vi "Android_Publisher_SM.vi"() -> ()   [LabVIEW 2015]
uses:
  <vilib>/daq.io/MQTT LabVIEW Client/Controls/Connection_Return_Codes.ctl
  Android_Data.ctl
  <vilib>/daq.io/MQTT LabVIEW Client/Controls/QoS.ctl
  <vilib>/daq.io/MQTT LabVIEW Client/Controls/Retain_Flag.ctl
  <vilib>/daq.io/MQTT LabVIEW Client/Controls/DUP_Flag.ctl
  Internet of Things Project/States.ctl
  <vilib>/Instr/_visa.llb/VISA Configure Serial Port (Instr).vi
  <vilib>/daq.io/MQTT LabVIEW Client/MQTT_Functions.lvlib
panel:
  in  "Data":T1={"VISA resource name"="ASRL1::INSTR", "baud rate (9600)"=19200, "Client ID"="myRIO", "Topic"="android", "MQTT Broker"={"address (IP)"="52.37.169.179", "port"=1883}, "Publish Meta"={"QoS"=enum."At most once", "Retain"=FALSE, "DUP"=FALSE}, "TCP connection ID "=refnum, "Session Status"=""}
  out "error out":errorcluster
  out "Session Status":string
  out "Published Data":string[][](array[string])
  in  "Stop Button":bool
  out "Connection Status":T5=enum."Connection refused: not authorized"
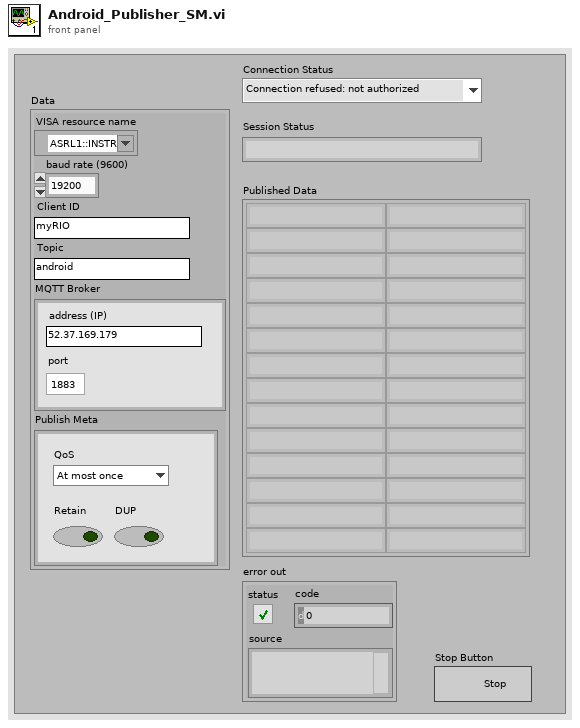
[diagram p1: front panel]
types:
  T1 = typedef "Android_Data.ctl" = cluster{"VISA resource name":refnum<visa-resource-name>, "baud rate (9600)":u32, "Client ID":string, "Topic":string, "MQTT Broker":cluster{"address (IP)":string, "port":u16}, "Publish Meta":cluster{"QoS":T2, "Retain":T3, "DUP":T4}, "TCP connection ID ":refnum<k5>, "Session Status":string}
  T2 = typedef "MQTT_Functions.lvlib/QoS.ctl" = enum8{"At most once", "At least once", "Exactly once", "Reserved"}
  T3 = typedef "MQTT_Functions.lvlib/Retain_Flag.ctl" = bool
  T4 = typedef "MQTT_Functions.lvlib/DUP_Flag.ctl" = bool
  T5 = typedef "MQTT_Functions.lvlib/Connection_Return_Codes.ctl" = enum16{"Connection accepted", "Connection refused: unacceptable protocol version", "Connection refused: identifier rejected", "Connection refused: Server unavailable", "Connection refused: bad user name or password", "Connection refused: not authorized"}
  T6 = typedef "States.ctl" = enum16{"Initialize", "TCP Connect", "Gather/Publish", "TCP Ping", "Exit/Disconnect"}
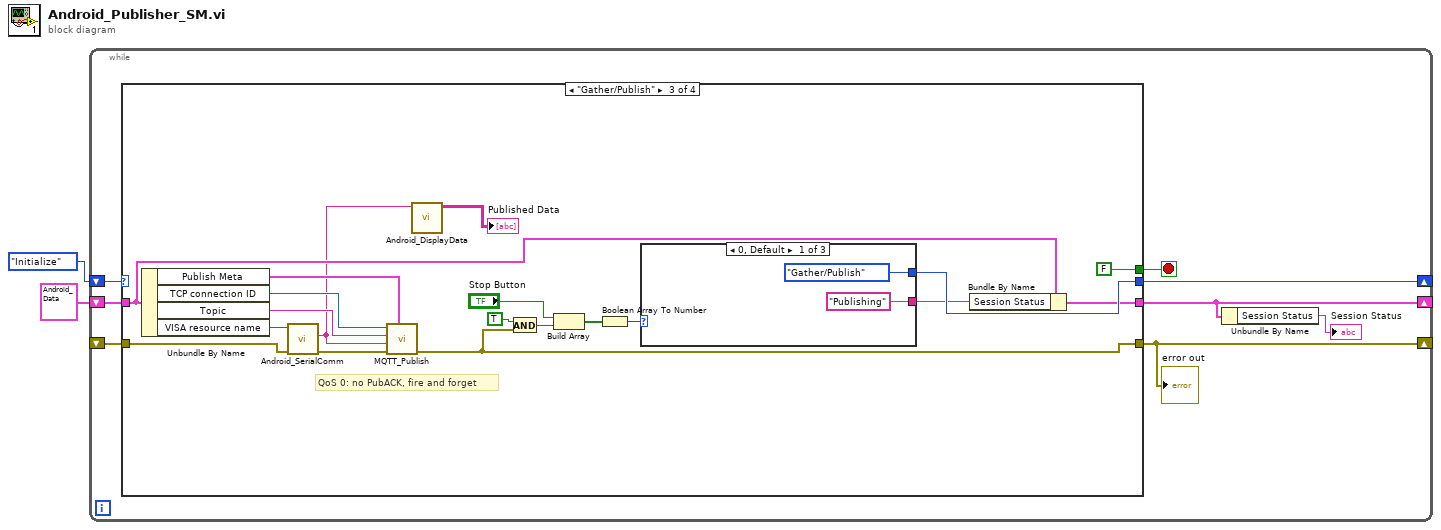
[diagram p0: block diagram]
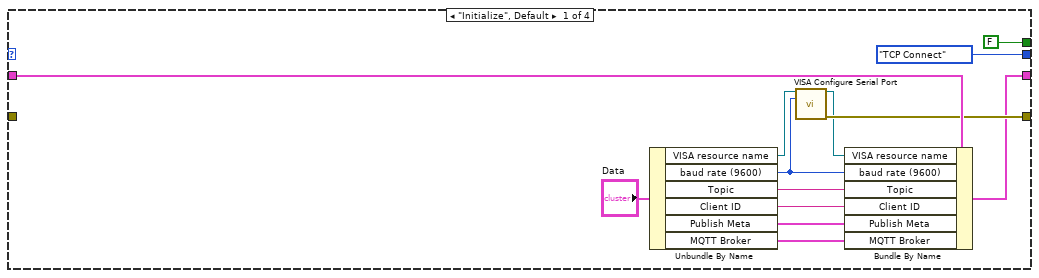
[diagram p2: hidden frame]
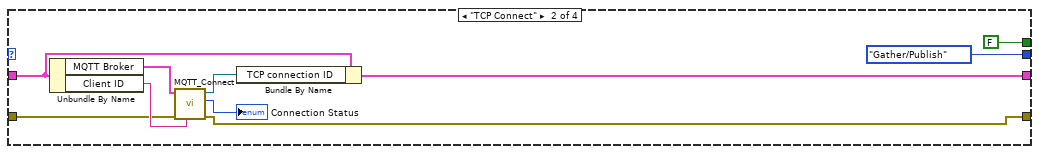
[diagram p3: hidden frame]
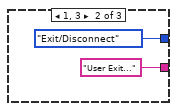
[diagram p4: hidden frame]
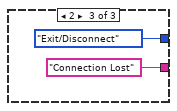
[diagram p5: hidden frame]
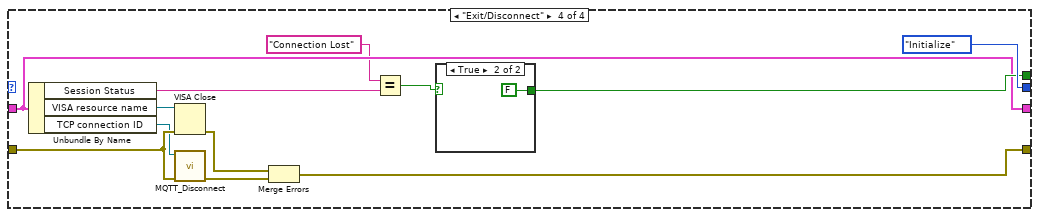
[diagram p6: hidden frame]
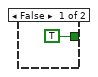
[diagram p7: hidden frame]
diagram:
  n1 = while {
    shift-right: [w10] -> _
    shift-left: States."Initialize" -> [w9]
    shift-right: [w5] -> _
    shift-left: T1 {"VISA resource name"="ASRL1::INSTR", "baud rate (9600)"=19200, "Client ID"="myRIO", "Topic"="data", "MQTT Broker"={"address (IP)"="52.37.169.179", "port"=1883}, "Publish Meta"={"QoS"=enum."At most once", "Retain"=FALSE, "DUP"=FALSE}, "TCP connection ID "=refnum, "Session Status"=""} ("Data") -> [w8]
    shift-right: [w3] -> _
    shift-left: _ -> [w7]
    stop <- w6 stop-if-true
    n2 = case shown="\"Gather/Publish\"" w9 {
      tunnel: [States."TCP Connect" States."Gather/Publish" w50 States."Initialize"] -> w10
      tunnel: w8 -> [w22 w28 w48 w63]
      tunnel: [w15 w26 w47 w63] -> w5
      tunnel: [w17 w30 w45 w59] -> w3
      tunnel: w7 -> [_ w25 w38 w69]
      tunnel: [FALSE FALSE FALSE w64] -> w6
      frame "Initialize", Default {
        n3 = Unbundle By Name("Data") -> ("VISA resource name"=w13:refnum<visa-resource-name>, "baud rate (9600)"=w11:u32, "Topic"=w18:string, "Client ID"=w19:string, "Publish Meta"=w20:cluster{"QoS":T2, "Retain":T3, "DUP":T4}, "MQTT Broker"=w21:cluster{"address (IP)":string, "port":u16})
        n4 = call-poly "VISA Configure Serial Port"("VISA resource name"=w13, "baud rate (9600)"=w11) -> ("VISA resource name out"=w12:refnum<visa-resource-name>, "error out"=w17:errorcluster)  [unwired: 12 in]
        n5 = Bundle By Name(cluster=w22, "VISA resource name"=w12, "baud rate (9600)"=w11, "Topic"=w18, "Client ID"=w19, "Publish Meta"=w20, "MQTT Broker"=w21) -> (w15:T1)
      }
      frame "TCP Connect" {
        n6 = Unbundle By Name(w28) -> ("MQTT Broker"=w32:cluster{"address (IP)":string, "port":u16}, "Client ID"=w31:string)
        n7 = call <vilib>:"MQTT_Connect.vi"("Client ID"=w31, "error in (no error)"=w25, "MQTT Broker"=w32) -> ("error out"=w30:errorcluster, "Connection Status"=→"Connection Status":T5, "connection ID out"=w27:refnum<k5>)  [unwired: 6 in]
        n8 = Bundle By Name(cluster=w28, "TCP connection ID"=w27) -> (w26:T1)
      }
      frame "Gather/Publish" {
        # "QoS 0: no PubACK, fire and forget"
        n9 = Unbundle By Name(w48) -> ("Publish Meta"=w52:cluster{"QoS":T2, "Retain":T3, "DUP":T4}, "TCP connection ID"=w39:refnum<k5>, "Topic"=w51:string, "VISA resource name"=w37:refnum<visa-resource-name>)
        n10 = call "Android_SerialComm.vi"("error in (no error)"=w38, "VISA Refnum in"=w37) -> ("error out"=w36:errorcluster, "Read Buffer"=w34:string)  [unwired: 7 in, 1 out]
        n11 = call <vilib>:"MQTT_Publish.vi"("Publish Meta"=w52, "error in (no error)"=w36, "Message to be published"=w34, "Topic"=w51, "connection ID"=w39) -> ("error out"=w45:errorcluster)  [unwired: 5 in, 1 out]
        n12 = call "Android_DisplayData.vi"("CSV Input"=w34) -> ("Published Data"=→"Published Data":string[][])  [unwired: 10 in]
        n13 = And(x=TRUE, y=w45) -> (x .and. y?=w40:bool)
        n14 = Build Array("Stop Button", w40) -> (w43:bool[])
        n15 = Boolean Array To Number(Boolean array=w43) -> (number=w42:u32)
        n16 = case shown="0, Default" w42 {
          tunnel: [States."Gather/Publish" States."Exit/Disconnect" States."Exit/Disconnect"] -> w50
          tunnel: ["Publishing" ("Session Status") "User Exit..." ("Session Status") "Connection Lost" ("Session Status")] -> w41
          frame 0, Default {
          }
          frame 1, 3 {
          }
          frame 2 {
          }
        }
        n17 = Bundle By Name(cluster=w48, "Session Status"=w41) -> (w47:T1)
      }
      frame "Exit/Disconnect" {
        n18 = Unbundle By Name(w63) -> ("Session Status"=w60:string, "VISA resource name"=w70:refnum<visa-resource-name>, "TCP connection ID"=w66:refnum<k5>)
        n19 = VISA Close(VISA resource name=w70, error in (no error)=w69) -> (error out=w67:errorcluster)
        n20 = call <vilib>:"MQTT_Disconnect.vi"("error in (no error)"=w69, "connection ID"=w66) -> ("error out"=w68:errorcluster)  [unwired: 9 in]
        n21 = Merge Errors(w67, w68) -> (w59:errorcluster)
        n22 = Equal?(x="Connection Lost" ("Session Status"), y=w60) -> (x = y?=w61:bool)
        n23 = case shown="True" w61 {
          tunnel: [TRUE FALSE] -> w64
          frame False {
          }
          frame True {
          }
        }
      }
    }
    "error out" <- w3
    n24 = Unbundle By Name(w5) -> ("Session Status"=→"Session Status":string)
  }
